vi "RandomizeIRL.vi"(11 "Difficulty":string) -> (3 "appended array 2":string[](array[string]))   [LabVIEW 2019]
doc: "Create an array of random moves to shuffle the cube"
uses:
  <vilib>/numeric/Random Number (Range) U64.vi
  <vilib>/numeric/sub_Random U32.vi
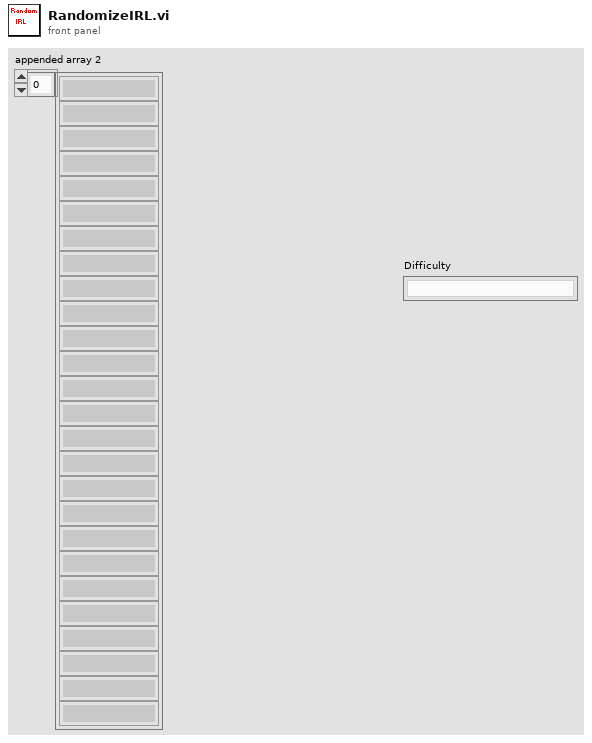
[diagram p1: front panel]
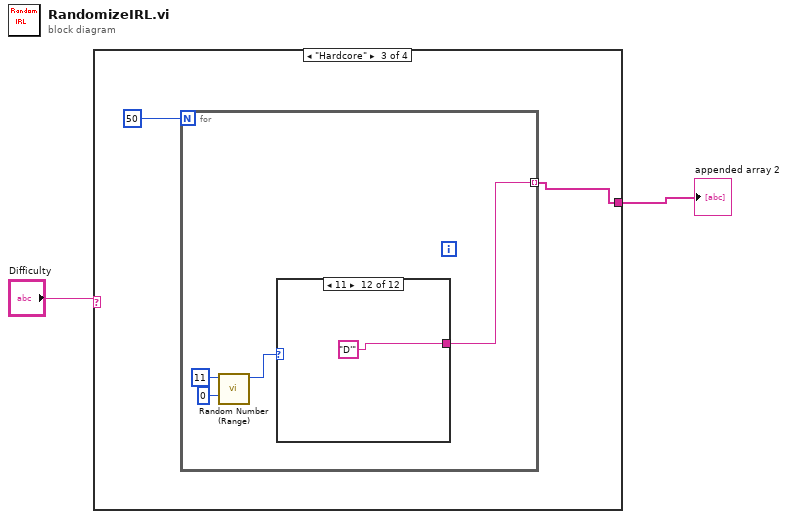
[diagram p0: block diagram]
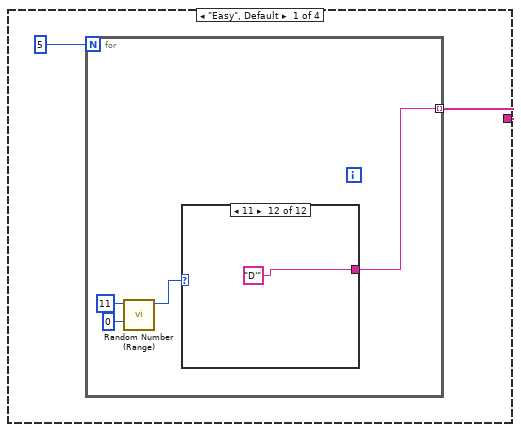
[diagram p2: hidden frame]
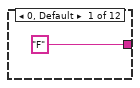
[diagram p3: hidden frame]
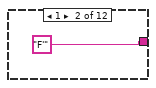
[diagram p4: hidden frame]
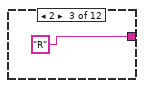
[diagram p5: hidden frame]
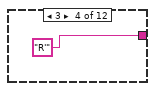
[diagram p6: hidden frame]
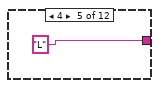
[diagram p7: hidden frame]
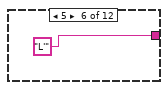
[diagram p8: hidden frame]
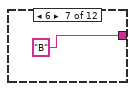
[diagram p9: hidden frame]
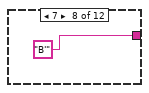
[diagram p10: hidden frame]
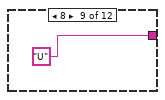
[diagram p11: hidden frame]
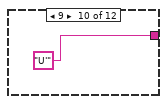
[diagram p12: hidden frame]
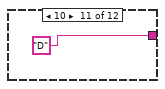
[diagram p13: hidden frame]
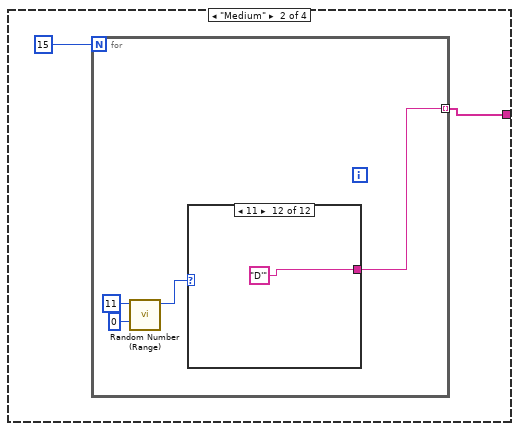
[diagram p14: hidden frame]
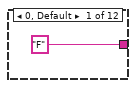
[diagram p15: hidden frame]
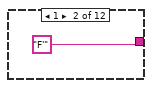
[diagram p16: hidden frame]
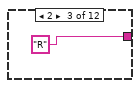
[diagram p17: hidden frame]
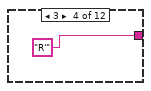
[diagram p18: hidden frame]
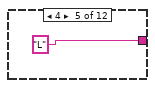
[diagram p19: hidden frame]
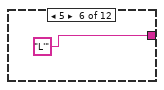
[diagram p20: hidden frame]
diagram:
  n1 = case shown="\"Hardcore\"" "Difficulty" {
    tunnel: [w3 w21 w39 w57] -> w1
    frame "Easy", Default {
      n2 = for {
        N: 5 -> [_]
        tunnel: [w5] -> w3 mode=indexing
        n3 = call-poly <vilib>:"Random Number (Range).vi"("lower bound (0)"=u64 0, "upper bound (100)"=u64 11) -> ("number"=w8:u64)  [unwired: 9 in]
        n4 = case shown="11" w8 {
          tunnel: ["F" "F'" "R" "R'" "L" "L'" "B" "B'" "U" "U'" "D" "D'"] -> w5
          frame 0, Default {
          }
          frame 1 {
          }
          frame 2 {
          }
          frame 3 {
          }
          frame 4 {
          }
          frame 5 {
          }
          frame 6 {
          }
          frame 7 {
          }
          frame 8 {
          }
          frame 9 {
          }
          frame 10 {
          }
          frame 11 {
          }
        }
      }
    }
    frame "Medium" {
      n5 = for {
        N: 15 -> [_]
        tunnel: [w23] -> w21 mode=indexing
        n6 = call-poly <vilib>:"Random Number (Range).vi"("lower bound (0)"=u64 0, "upper bound (100)"=u64 11) -> ("number"=w26:u64)  [unwired: 9 in]
        n7 = case shown="11" w26 {
          tunnel: ["F" "F'" "R" "R'" "L" "L'" "B" "B'" "U" "U'" "D" "D'"] -> w23
          frame 0, Default {
          }
          frame 1 {
          }
          frame 2 {
          }
          frame 3 {
          }
          frame 4 {
          }
          frame 5 {
          }
          frame 6 {
          }
          frame 7 {
          }
          frame 8 {
          }
          frame 9 {
          }
          frame 10 {
          }
          frame 11 {
          }
        }
      }
    }
    frame "Hardcore" {
      n8 = for {
        N: 50 -> [_]
        tunnel: [w41] -> w39 mode=indexing
        n9 = call-poly <vilib>:"Random Number (Range).vi"("lower bound (0)"=u64 0, "upper bound (100)"=u64 11) -> ("number"=w44:u64)  [unwired: 9 in]
        n10 = case shown="11" w44 {
          tunnel: ["F" "F'" "R" "R'" "L" "L'" "B" "B'" "U" "U'" "D" "D'"] -> w41
          frame 0, Default {
          }
          frame 1 {
          }
          frame 2 {
          }
          frame 3 {
          }
          frame 4 {
          }
          frame 5 {
          }
          frame 6 {
          }
          frame 7 {
          }
          frame 8 {
          }
          frame 9 {
          }
          frame 10 {
          }
          frame 11 {
          }
        }
      }
    }
    frame "Hard" {
      n11 = for {
        N: 25 -> [_]
        tunnel: [w59] -> w57 mode=indexing
        n12 = call-poly <vilib>:"Random Number (Range).vi"("lower bound (0)"=u64 0, "upper bound (100)"=u64 11) -> ("number"=w62:u64)  [unwired: 9 in]
        n13 = case shown="11" w62 {
          tunnel: ["F" "F'" "R" "R'" "L" "L'" "B" "B'" "U" "U'" "D" "D'"] -> w59
          frame 0, Default {
          }
          frame 1 {
          }
          frame 2 {
          }
          frame 3 {
          }
          frame 4 {
          }
          frame 5 {
          }
          frame 6 {
          }
          frame 7 {
          }
          frame 8 {
          }
          frame 9 {
          }
          frame 10 {
          }
          frame 11 {
          }
        }
      }
    }
  }
  "appended array 2" <- w1
